vi "get_name.vi"(8 "error in (no error)":errorcluster, 11 "VINode in":refnum<class "HierarchyNode.lvclass">) -> (0 "error out":errorcluster, 2 "Name":string, 3 "VINode out":refnum<class "HierarchyNode.lvclass">)   [LabVIEW 2020, in "vi-hierarchy.lvlib" / "HierarchyNode.lvclass"]
uses:
  HierarchyNode.lvclass
  HierarchyNode.lvclass/HierarchyNode.ctl
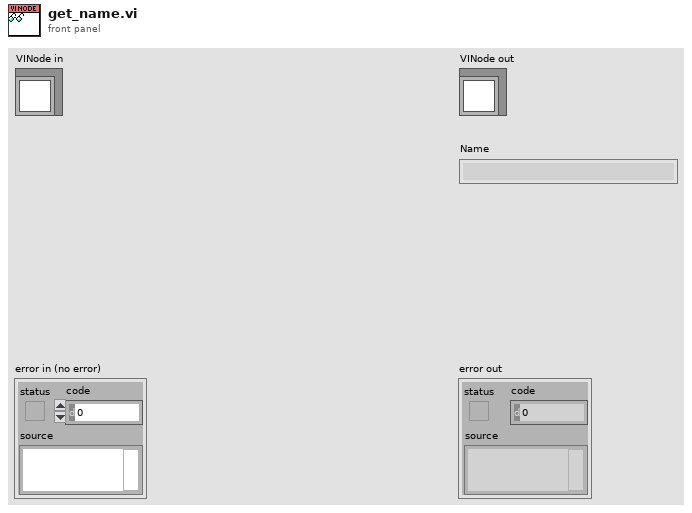
[diagram p1: front panel]
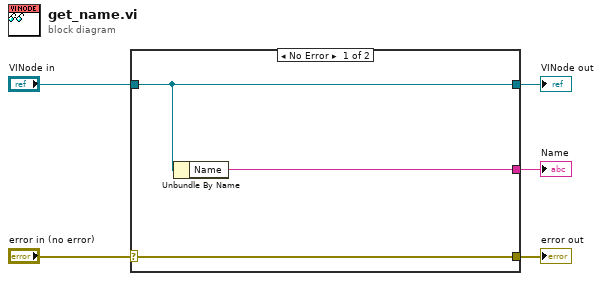
[diagram p0: block diagram]
diagram:
  n1 = case shown="No Error" "error in (no error)" {
    selector: "error in (no error)" -> [w8 w9]
    tunnel: [w8 w9] -> w4
    tunnel: [w7 w10] -> w2
    tunnel: "VINode in" -> [w7 w10]
    tunnel: [w6 _] -> w1
    frame No Error {
      n2 = Unbundle By Name(w7) -> ("Name"=w6:string)
    }
    frame Error {
    }
  }
  "error out" <- w4
  "VINode out" <- w2
  "Name" <- w1
